vi "Timestamp String to LV Timestamp Poly.vi"   [LabVIEW 2018]
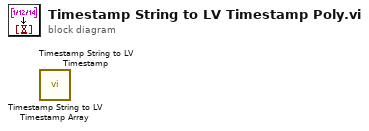
[diagram p0: block diagram]
diagram:
  n1 = call "Timestamp String to LV Timestamp Array.vi"() -> ()  [unwired: 1 in, 2 out]
  n2 = call "Timestamp String to LV Timestamp.vi"() -> ()  [unwired: 1 in, 2 out]
